vi "Shutdown.vi"   [LabVIEW 2014]
uses:
  <userlib>/Nanonis Prog Interface V5/Nanonis Prog Interface.lvlib
types:
  T1 = enum8{"Group 1", "Group 2", "Group 3", "Group 4", "Group 5", "Group 6"}
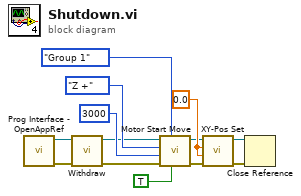
[diagram p0: block diagram]
diagram:
  w11 = sgl 0.0 ("X (m)")
  n1 = call <userlib>:"Prog Interface - OpenAppRef.vi"() -> ("Error out"=w13:errorcluster, "Application reference"=w12:refnum<vi>)  [unwired: 6 in]
  n2 = call <userlib>:"Withdraw.vi"("Error in (no error)"=w13, "Application ref in"=w12) -> ("Error out"=w1:errorcluster, "Application ref out"=w2:refnum<vi>)  [unwired: 8 in]
  n3 = call <userlib>:"Motor Start Move.vi"("Wait until finished? (F)"=TRUE, "Group"=T1."Group 1", "Error in (no error)"=w1, "Number of steps"=u16 3000, "Direction"=enum16{"X +", "X -", "Y +", "Y -", "Z +", "Z -"}."Z +", "Application ref in"=w2) -> ("Error out"=w4:errorcluster, "Application ref out"=w3:refnum<vi>)  [unwired: 3 in]
  n4 = call <userlib>:"XY-Pos Set.vi"("error in (no error)"=w4, "Y (m)"=w11, "X (m)"=w11, "Application ref in"=w3) -> ("error out"=w5:errorcluster, "Application ref out"=w6:refnum<vi>)  [unwired: 4 in]
  n5 = Close Reference(reference=w6, error in (no error)=w5) -> ()  [unwired: 1 out]
